vi "H-MEDI PatientsList.vi"() -> ()   [LabVIEW 2019]
uses:
  03_Home/controller/logoutBtn.ctl
  03_Home/controller/exitBtn.ctl
  <vilib>/Utility/miscctls.llb/LVPointTypeDef.ctl
  03_Home/controller/pannelState.ctl
  globalValue.vi
panel:
  in  "backPage":bool
  out "totalCount":string
  in  "totalPage":i8
  in  "crrentPage":i8
  in  "leftBtn":bool
  in  "rightBtn":bool
  in  "btnGroup":T1
  out "userList":i32(listbox)
  in  "searchBtn":bool
  in  "searchForm":string
  in  "Help Button":bool
  in  "LogOut Button":T2
  in  "Exit Button":T3
  out "userNm":string
  # "/"
  # "|"
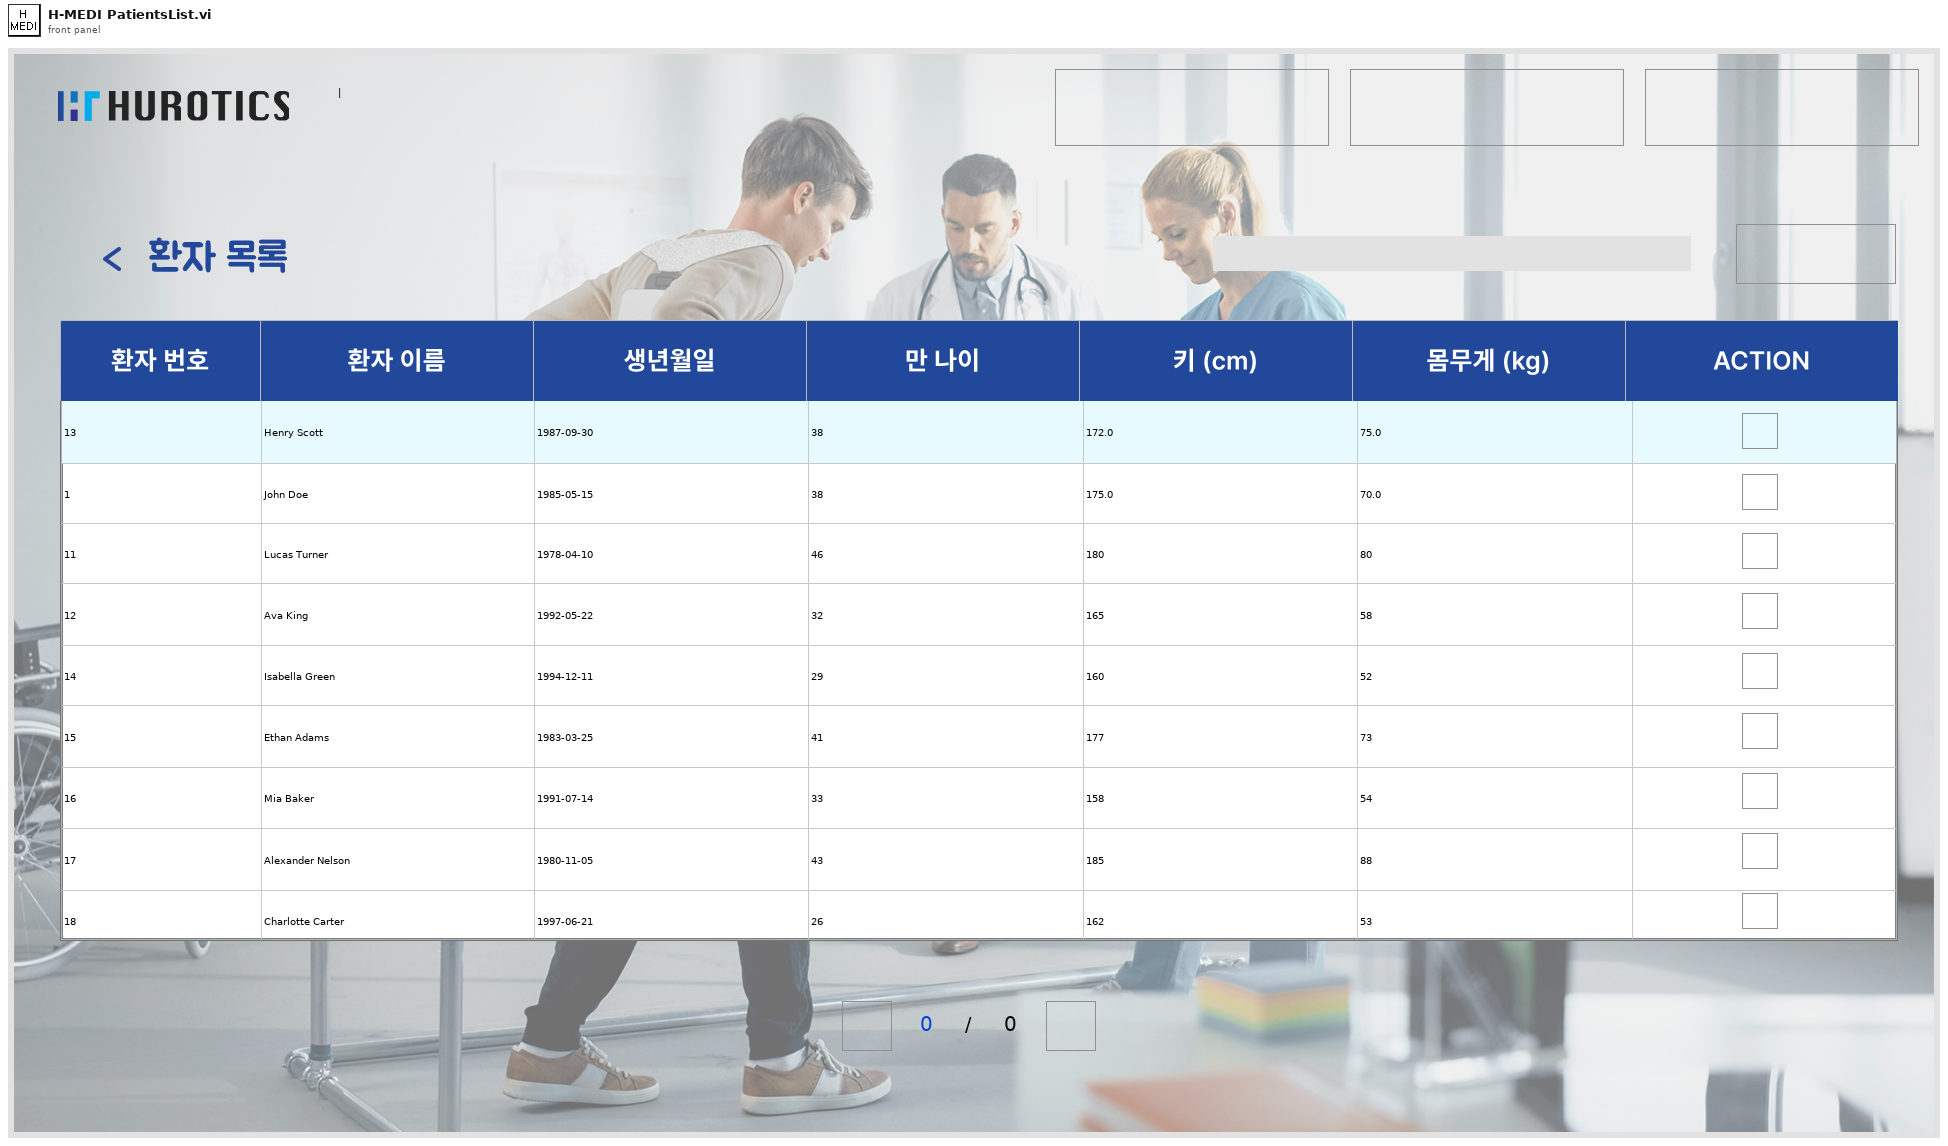
[diagram p1: front panel]
types:
  T1 = cluster{"불리언":bool, "불리언 2":bool, "불리언 3":bool, "불리언 4":bool, "불리언 5":bool, "불리언 6":bool, "불리언 7":bool, "불리언 8":bool, "불리언 9":bool}
  T2 = typedef "logoutBtn.ctl" = bool
  T3 = typedef "exitBtn.ctl" = bool
  T4 = typedef "LVPointTypeDef.ctl" = cluster{"Horizontal":i16, "Vertical":i16}
  T5 = enum16{"connection", "create", "getReadList", "getRead", "getCount", "update", "delete", "close"}
  T6 = typedef "pannelState.ctl" = enum16{"Init", "LogIn", "SignUpView", "Home", "Management_patientList", "Management_patientTrashtList", "Management_patientCreate", "Management_patientUpdate", "Management_patientTraining", "Management_patientTrainingDetail", "H-MEDI PatientList", "H-MEDI HardwareCtl", "Adjust", "FineTuning", "UserList", "UserDetail", "Exit"}
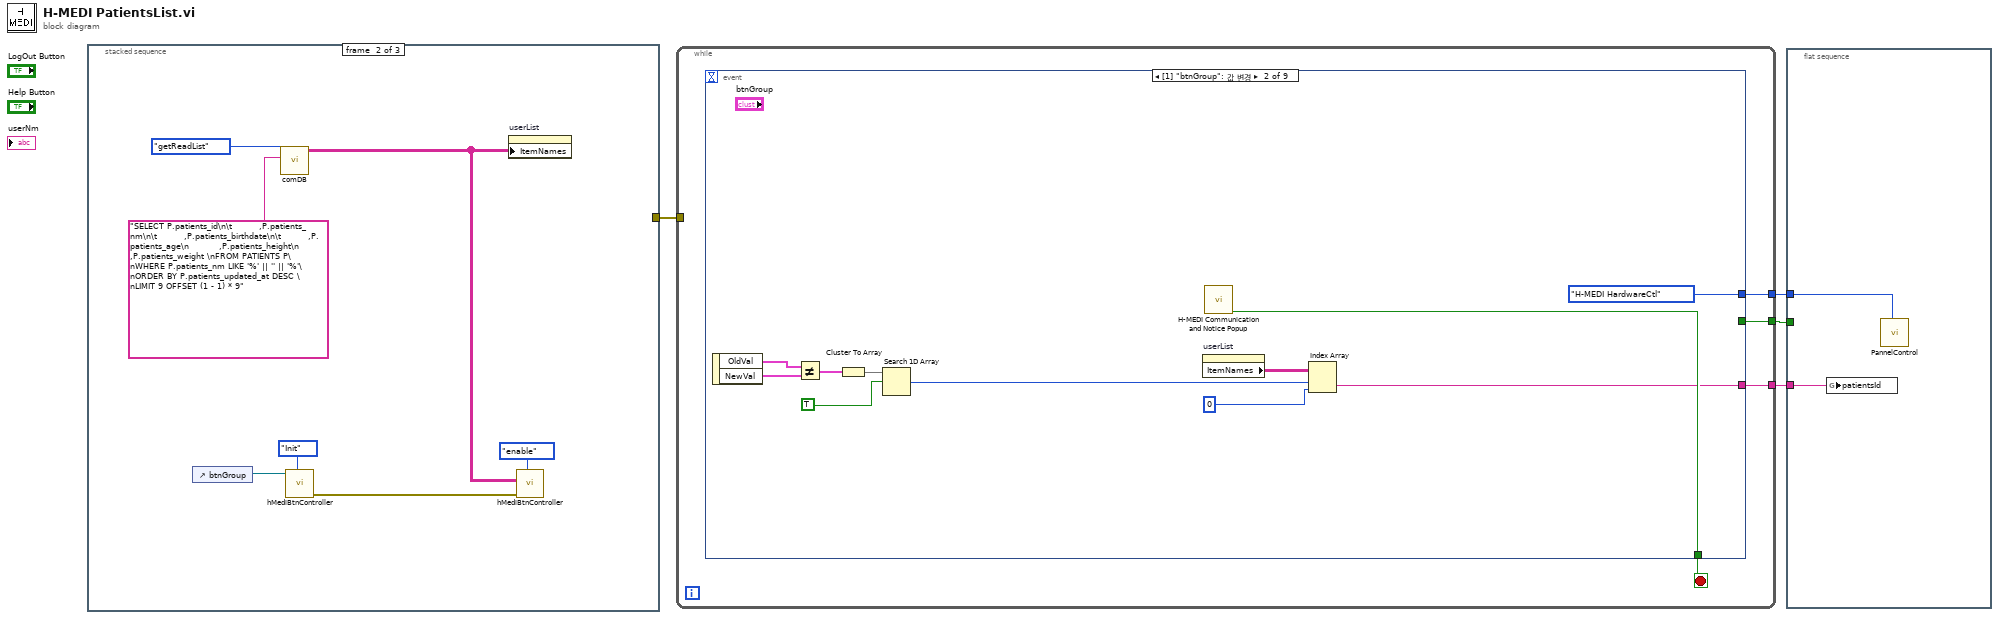
[diagram p0: block diagram]
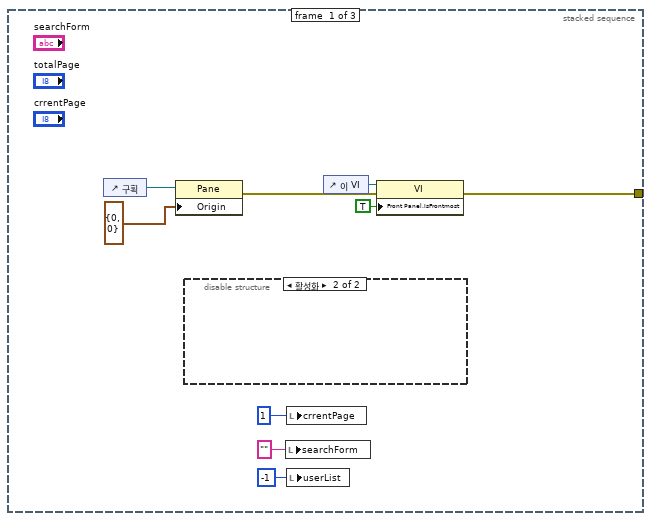
[diagram p2: hidden frame]
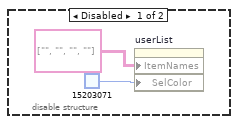
[diagram p3: hidden frame]
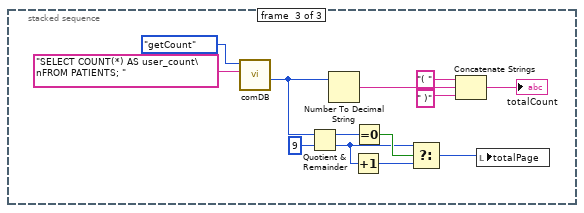
[diagram p4: hidden frame]
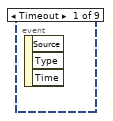
[diagram p5: hidden frame]
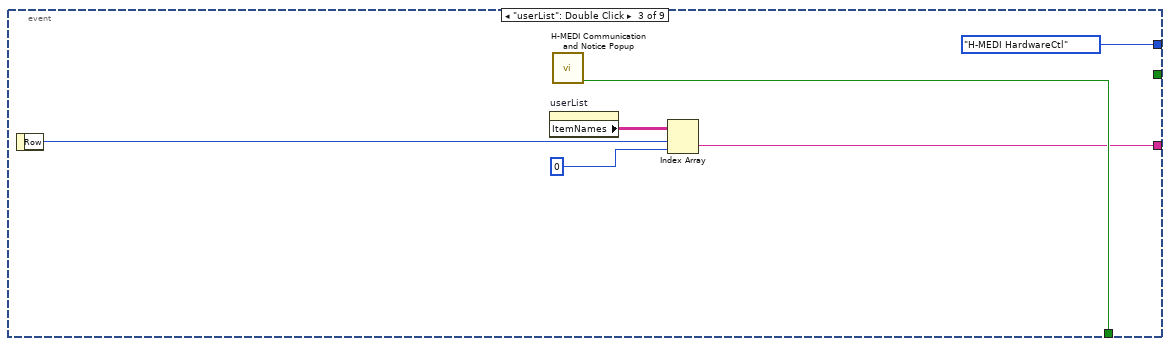
[diagram p6: hidden frame]
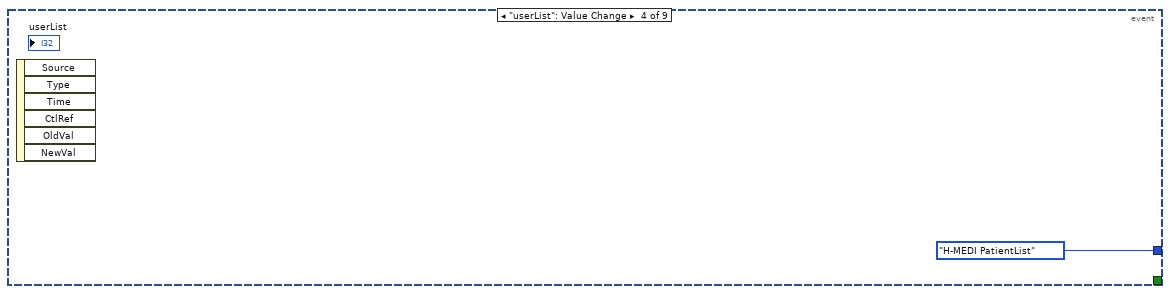
[diagram p7: hidden frame]
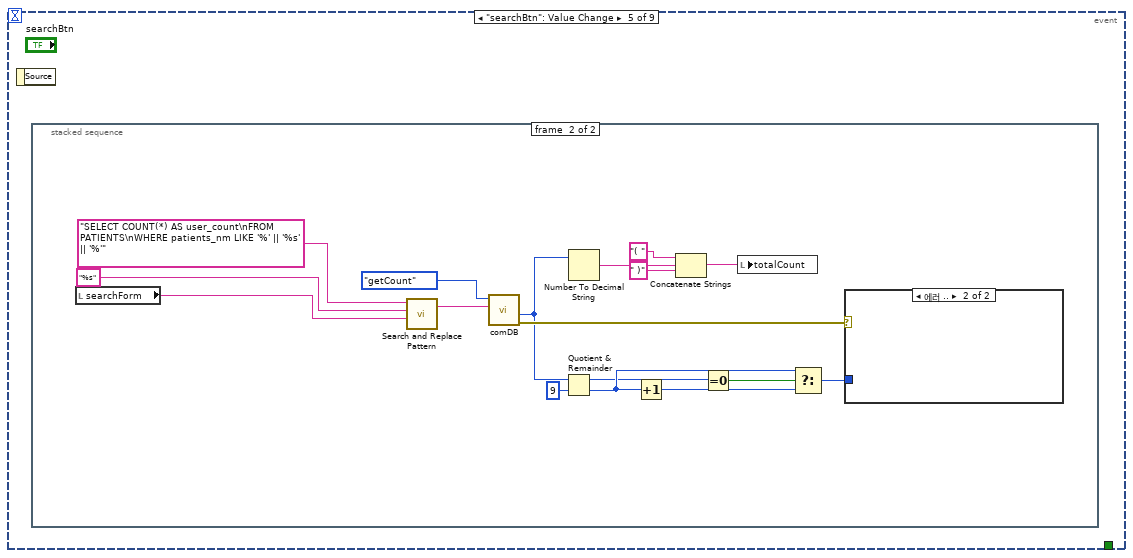
[diagram p8: hidden frame]
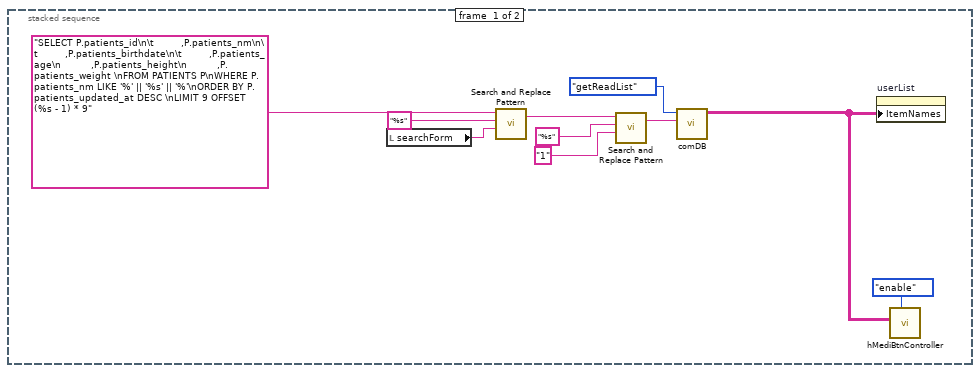
[diagram p9: hidden frame]
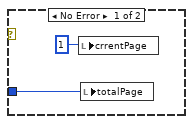
[diagram p10: hidden frame]
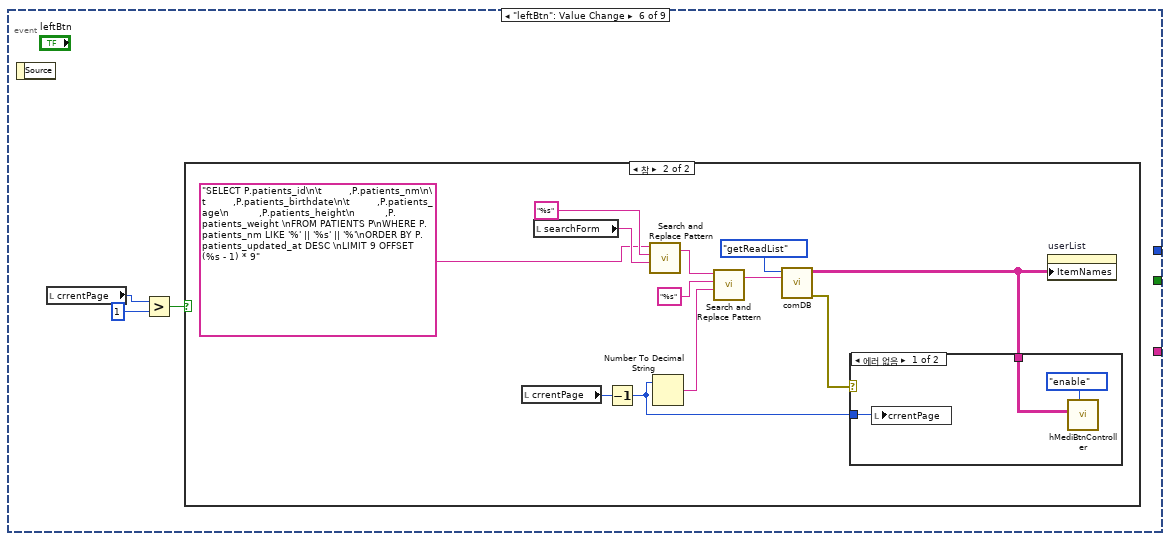
[diagram p11: hidden frame]
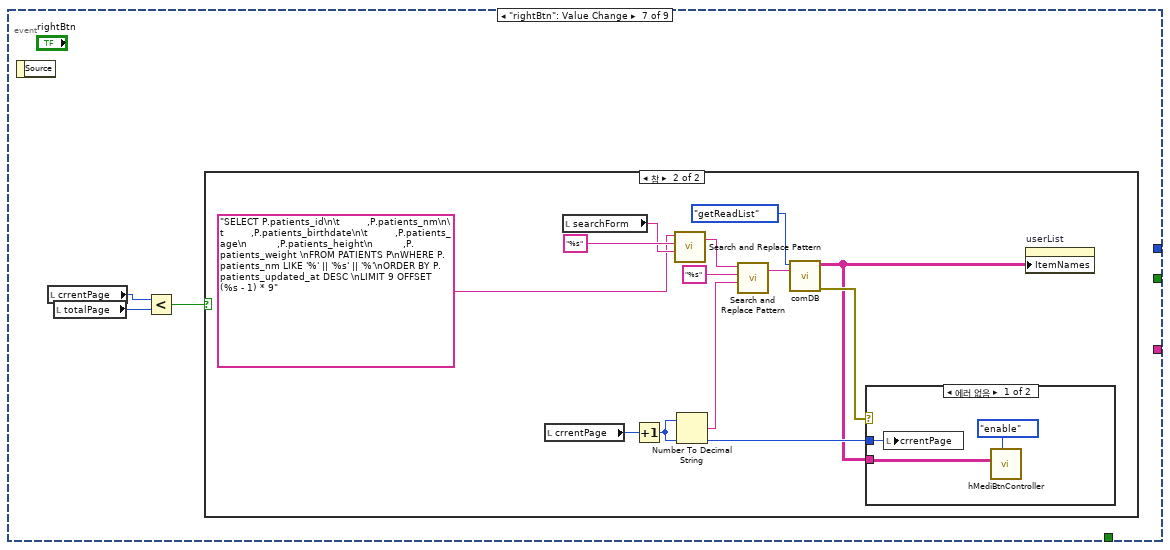
[diagram p14: hidden frame]
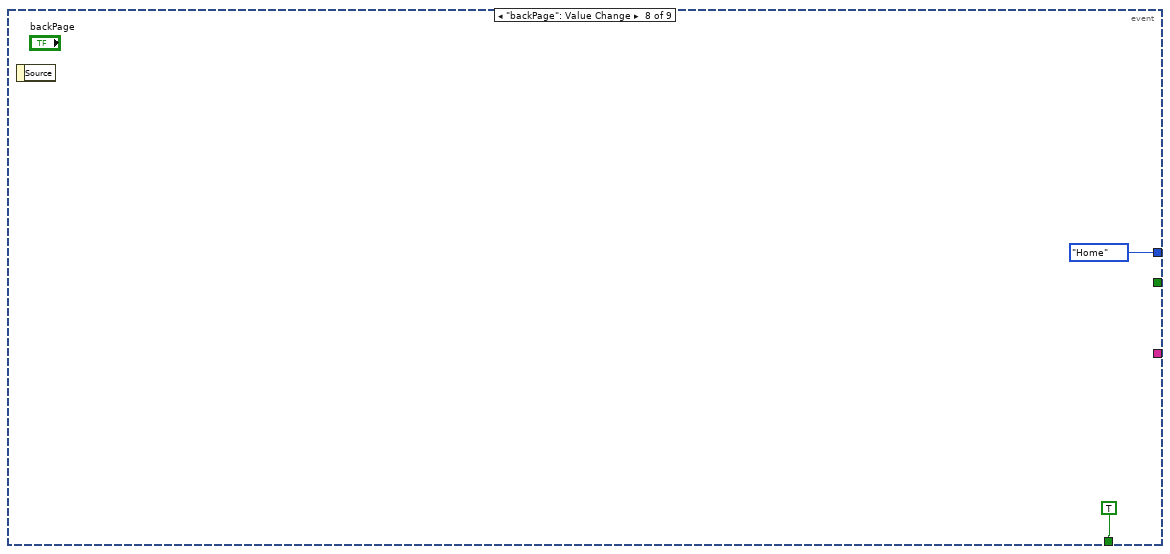
[diagram p17: hidden frame]
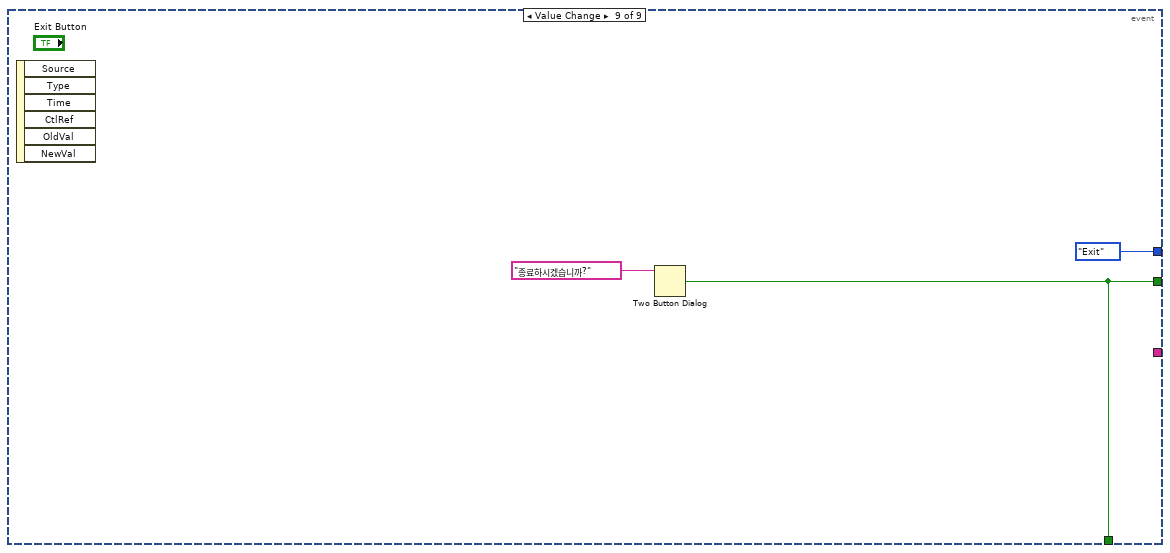
[diagram p18: hidden frame]
diagram:
  n1 = stacked-sequence {
    tunnel: [w5 _ _] -> w4
    frame #0 {
      n2 = control-ref of="구획"() -> (w11:refnum<vi>)
      n3 = property class="Pane"(reference=w11, "Origin"=T4 {"Horizontal"=0, "Vertical"=0} ("원점")) -> (error out=w9:errorcluster)  [unwired: 1 in, 1 out]
      n4 = disable-structure shown="활성화" {
        frame Disabled {
          n5 = property on="userList" class="MCListbox (엄격한)"("ItemNames"=string[][] [["", ""], ["", ""]], "SelColor"=u32 15203071 ("선택 색")) -> ()  [unwired: 2 in, 2 out]
        }
        frame Enabled {
        }
      }
      n6 = local write "searchForm"("" ("searchForm")) -> ()
      n7 = local write "crrentPage"(i8 1 ("crrentPage")) -> ()
      n8 = local write "userList"(-1 ("userList")) -> ()
      n9 = control-ref of="이 VI"() -> (w13:refnum<vi>)
      n10 = property class="VI"(reference=w13, error in=w9, "Front Panel.IsFrontmost"=TRUE ("프런트패널 윈도우:맨 앞으로")) -> (error out=w5:errorcluster)  [unwired: 1 out]
    }
    frame #1 {
      n11 = control-ref of="btnGroup"() -> (w16:refnum<vi>)
      n12 = call "comDB.vi"("Query"="SELECT P.patients_id\n\t         ,P.patients_nm\n\t         ,P.patients_birthdate\n\t         ,P.patients_age\n          ,P.patients_height\n          ,P.patients_weight \nFROM PATIENTS P\nWHERE P.patients_nm LIKE '%' || '' || '%'\nORDER BY P.patients_updated_at DESC \nLIMIT 9 OFFSET (1 - 1) * 9", "State"=T5."getReadList") -> ("resultList"=w20:string[][])  [unwired: 5 in, 3 out]
      n13 = call "hMediBtnController.vi"("state"=enum16{"Init", "enable"}."Init", "btnGroup"=w16) -> ("error out"=w19:errorcluster)  [unwired: 9 in]
      n14 = property on="userList" class="MCListbox (엄격한)"("ItemNames"=w20) -> ()  [unwired: 2 in, 2 out]
      n15 = call "hMediBtnController.vi"("state"=enum16{"Init", "enable"}."enable", "error in (no error)"=w19, "2dArray"=w20) -> ()  [unwired: 8 in, 1 out]
    }
    frame #2 {
      n16 = call "comDB.vi"("Query"="SELECT COUNT(*) AS user_count\nFROM PATIENTS; ", "State"=T5."getCount") -> ("count"=w27:i64)  [unwired: 5 in, 3 out]
      n17 = Quotient & Remainder(x=w27, y=i64 9) -> (x-y*floor(x/y)=w24:i64, floor(x/y)=w23:i64)
      n18 = Number To Decimal String(number=w27) -> (decimal integer string=w31:string)  [unwired: 1 in]
      n19 = Increment(x=w23) -> (x+1=w28:i64)
      n20 = Equal To 0?(x=w24) -> (x = 0?=w25:bool)
      n21 = Select(t=w23, s=w25, f=w28) -> (s? t:f=w26:i64)
      n22 = Concatenate Strings("( ", w31, " )") -> (→"totalCount":string)
      n23 = local write "totalPage"(w26) -> ()
    }
  }
  n24 = while {
    tunnel: w4 -> [_]
    tunnel: [w38] -> w3
    tunnel: [w37] -> w2
    tunnel: [w36] -> w1
    stop <- w39 stop-if-true
    n25 = event shown="[1] \"btnGroup\": 값 변경" {
      selector: _ -> [_ _ _ _ _ _ _ _ _]
      dyn-events: _ -> [_ _ _ _ _ _ _ _ _]
      timeout: _ -> [_ _ _ _ _ _ _ _ _]
      tunnel: [_ w50 w56 _ _ _ _ TRUE w126] -> w39
      tunnel: [_ _ _ _ _ _ _ _ w126] -> w38
      tunnel: [_ pannelState."H-MEDI HardwareCtl" ("State") pannelState."H-MEDI HardwareCtl" ("State") pannelState."H-MEDI PatientList" ("State") _ _ _ pannelState."Home" ("State") pannelState."Exit" ("State")] -> w37
      tunnel: [_ w46 w51 _ _ _ _ _ _] -> w36
      event Timeout {
        n26 = event-data() -> ()  [unwired: 1 in, 3 out]
      }
      event "btnGroup": Value Change {
        n27 = event-data() -> ("OldVal"=w45:T1, "NewVal"=w44:T1)  [unwired: 1 in]
        n28 = Not Equal?(x=w45, y=w44) -> (x != y?=w43:T1)
        n29 = Cluster To Array(cluster=w43) -> (array=w42:bool[])
        n30 = Search 1D Array(1D array=w42, element=TRUE) -> (index of element=w40:i32)  [unwired: 1 in]
        n31 = property on="userList" class="MCListbox (엄격한)"() -> ("ItemNames"=w48:string[][])  [unwired: 2 in, 2 out]
        n32 = call "H-MEDI Communication and Notice Popup.vi"() -> ("HW control on"=w50:bool)  [unwired: 11 in]
        n33 = Index Array(array=w48, index (row)=w40, index (col)=0 ("비활성화된 인덱스 (열)")) -> (element=w46:string)
      }
      event "userList": Double Click {
        n34 = event-data() -> ("Row"=w53:i32)  [unwired: 1 in]
        n35 = property on="userList" class="MCListbox (엄격한)"() -> ("ItemNames"=w54:string[][])  [unwired: 2 in, 2 out]
        n36 = call "H-MEDI Communication and Notice Popup.vi"() -> ("HW control on"=w56:bool)  [unwired: 11 in]
        n37 = Index Array(array=w54, index (row)=w53, index (col)=0 ("비활성화된 인덱스 (열)")) -> (element=w51:string)
      }
      event "userList": Value Change {
        n38 = event-data() -> ()  [unwired: 1 in, 6 out]
      }
      event "searchBtn": Value Change {
        n39 = event-data() -> ()  [unwired: 1 in, 1 out]
        n40 = stacked-sequence {
          frame #0 {
            n41 = local read "searchForm"() -> (w65:string)
            n42 = call <vilib>:"Search and Replace Pattern.vi"("string"="SELECT P.patients_id\n\t         ,P.patients_nm\n\t         ,P.patients_birthdate\n\t         ,P.patients_age\n          ,P.patients_height\n          ,P.patients_weight \nFROM PATIENTS P\nWHERE P.patients_nm LIKE '%' || '%s' || '%'\nORDER BY P.patients_updated_at DESC \nLIMIT 9 OFFSET (%s - 1) * 9" ("Query"), "regular expression (\"\")"="%s" ("regular expression (\"\")"), "replace string (\"\")"=w65) -> ("result string"=w64:string)  [unwired: 2 in, 1 out]
            n43 = call <vilib>:"Search and Replace Pattern.vi"("string"=w64, "regular expression (\"\")"="%s" ("regular expression (\"\")"), "replace string (\"\")"="1" ("regular expression (\"\")")) -> ("result string"=w61:string)  [unwired: 2 in, 1 out]
            n44 = call "comDB.vi"("Query"=w61, "State"=T5."getReadList") -> ("resultList"=w60:string[][])  [unwired: 5 in, 3 out]
            n45 = property on="userList" class="MCListbox (엄격한)"("ItemNames"=w60) -> ()  [unwired: 2 in, 2 out]
            n46 = call "hMediBtnController.vi"("state"=enum16{"Init", "enable"}."enable", "2dArray"=w60) -> ()  [unwired: 9 in, 1 out]
          }
          frame #1 {
            n47 = local read "searchForm"() -> (w84:string)
            n48 = call <vilib>:"Search and Replace Pattern.vi"("string"="SELECT COUNT(*) AS user_count\nFROM PATIENTS\nWHERE patients_nm LIKE '%' || '%s' || '%'" ("Query"), "regular expression (\"\")"="%s" ("regular expression (\"\")"), "replace string (\"\")"=w84) -> ("result string"=w81:string)  [unwired: 2 in, 1 out]
            n49 = call "comDB.vi"("Query"=w81, "State"=T5."getCount") -> ("error out"=w80:errorcluster, "count"=w74:i64)  [unwired: 5 in, 2 out]
            n50 = Quotient & Remainder(x=w74, y=i64 9) -> (x-y*floor(x/y)=w69:i64, floor(x/y)=w70:i64)
            n51 = Number To Decimal String(number=w74) -> (decimal integer string=w75:string)  [unwired: 1 in]
            n52 = Increment(x=w70) -> (x+1=w72:i64)
            n53 = Concatenate Strings("( ", w75, " )") -> (w76:string)
            n54 = Equal To 0?(x=w69) -> (x = 0?=w68:bool)
            n55 = local write "totalCount"(w76) -> ()
            n56 = Select(t=w70, s=w68, f=w72) -> (s? t:f=w71:i64)
            n57 = case shown="에러 .." w80 {
              tunnel: w71 -> [w85 _]
              frame No Error {
                n58 = local write "crrentPage"(i8 1 ("crrentPage")) -> ()
                n59 = local write "totalPage"(w85) -> ()
              }
              frame Error {
              }
            }
          }
        }
      }
      event "leftBtn": Value Change {
        n60 = event-data() -> ()  [unwired: 1 in, 1 out]
        n61 = local read "crrentPage"() -> (w87:i8)
        n62 = Greater?(x=w87, y=1) -> (0:w89:bool)
        n63 = case shown="참" w89 {
          frame False {
          }
          frame True {
            n64 = local read "crrentPage"() -> (w101:i8)
            n65 = local read "searchForm"() -> (w94:string)
            n66 = Decrement(x=w101) -> (x-1=w95:i8)
            n67 = call <vilib>:"Search and Replace Pattern.vi"("string"="SELECT P.patients_id\n\t         ,P.patients_nm\n\t         ,P.patients_birthdate\n\t         ,P.patients_age\n          ,P.patients_height\n          ,P.patients_weight \nFROM PATIENTS P\nWHERE P.patients_nm LIKE '%' || '%s' || '%'\nORDER BY P.patients_updated_at DESC \nLIMIT 9 OFFSET (%s - 1) * 9" ("Query"), "regular expression (\"\")"="%s" ("regular expression (\"\")"), "replace string (\"\")"=w94) -> ("result string"=w92:string)  [unwired: 2 in, 1 out]
            n68 = Number To Decimal String(number=w95) -> (decimal integer string=w99:string)  [unwired: 1 in]
            n69 = call <vilib>:"Search and Replace Pattern.vi"("string"=w92, "regular expression (\"\")"="%s" ("regular expression (\"\")"), "replace string (\"\")"=w99) -> ("result string"=w98:string)  [unwired: 2 in, 1 out]
            n70 = call "comDB.vi"("Query"=w98, "State"=T5."getReadList") -> ("error out"=w96:errorcluster, "resultList"=w91:string[][])  [unwired: 5 in, 2 out]
            n71 = case shown="에러 없음" w96 {
              tunnel: w95 -> [w104 _]
              tunnel: w91 -> [w103 _]
              frame No Error {
                n72 = local write "crrentPage"(w104) -> ()
                n73 = call "hMediBtnController.vi"("state"=enum16{"Init", "enable"}."enable", "2dArray"=w103) -> ()  [unwired: 9 in, 1 out]
              }
              frame Error {
              }
            }
            n74 = property on="userList" class="MCListbox (엄격한)"("ItemNames"=w91) -> ()  [unwired: 2 in, 2 out]
          }
        }
      }
      event "rightBtn": Value Change {
        n75 = event-data() -> ()  [unwired: 1 in, 1 out]
        n76 = local read "crrentPage"() -> (w106:i8)
        n77 = local read "totalPage"() -> (w105:i8)
        n78 = Less?(x=w106, y=w105) -> (x < y?=w107:bool)
        n79 = case shown="참" w107 {
          frame False {
          }
          frame True {
            n80 = local read "crrentPage"() -> (w119:i8)
            n81 = local read "searchForm"() -> (w111:string)
            n82 = Increment(x=w119) -> (x+1=w113:i8)
            n83 = call <vilib>:"Search and Replace Pattern.vi"("string"="SELECT P.patients_id\n\t         ,P.patients_nm\n\t         ,P.patients_birthdate\n\t         ,P.patients_age\n          ,P.patients_height\n          ,P.patients_weight \nFROM PATIENTS P\nWHERE P.patients_nm LIKE '%' || '%s' || '%'\nORDER BY P.patients_updated_at DESC \nLIMIT 9 OFFSET (%s - 1) * 9" ("Query"), "regular expression (\"\")"="%s" ("regular expression (\"\")"), "replace string (\"\")"=w111) -> ("result string"=w110:string)  [unwired: 2 in, 1 out]
            n84 = Number To Decimal String(number=w113) -> (decimal integer string=w117:string)  [unwired: 1 in]
            n85 = call <vilib>:"Search and Replace Pattern.vi"("string"=w110, "regular expression (\"\")"="%s" ("regular expression (\"\")"), "replace string (\"\")"=w117) -> ("result string"=w116:string)  [unwired: 2 in, 1 out]
            n86 = call "comDB.vi"("Query"=w116, "State"=T5."getReadList") -> ("error out"=w114:errorcluster, "resultList"=w109:string[][])  [unwired: 5 in, 2 out]
            n87 = case shown="에러 없음" w114 {
              tunnel: w113 -> [w122 _]
              tunnel: w109 -> [w121 _]
              frame No Error {
                n88 = local write "crrentPage"(w122) -> ()
                n89 = call "hMediBtnController.vi"("state"=enum16{"Init", "enable"}."enable", "2dArray"=w121) -> ()  [unwired: 9 in, 1 out]
              }
              frame Error {
              }
            }
            n90 = property on="userList" class="MCListbox (엄격한)"("ItemNames"=w109) -> ()  [unwired: 2 in, 2 out]
          }
        }
      }
      event "backPage": Value Change {
        n91 = event-data() -> ()  [unwired: 1 in, 1 out]
      }
      event Value Change {
        n92 = event-data() -> ()  [unwired: 1 in, 6 out]
        n93 = Two Button Dialog(message="종료하시겠습니까?" ("메시지")) -> (T button?=w126:bool)  [unwired: 2 in]
      }
    }
  }
  n94 = flat-sequence {
    tunnel: w3 -> [_]
    tunnel: w2 -> [w129]
    tunnel: w1 -> [w128]
    frame #0 {
      n95 = global write "globalValue.vi" "patientsId"(w128) -> ()
      n96 = call "PannelControl.vi"("State"=w129) -> ()  [unwired: 10 in, 1 out]
    }
  }
